vi "子VI-信息说明界面.vi"() -> ()   [LabVIEW 2018]
panel:
  in  "确认":bool
  out "使用说明":string
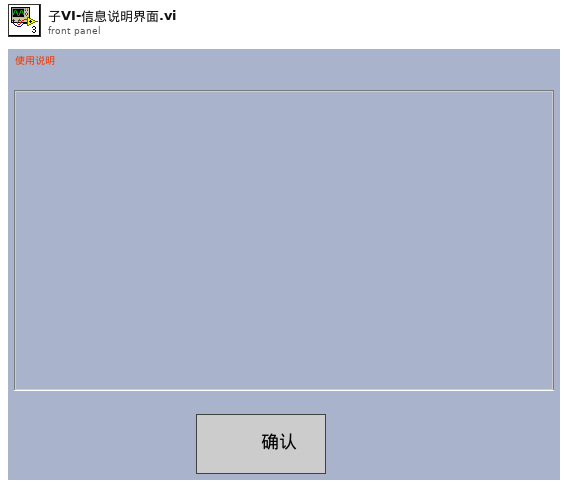
[diagram p1: front panel]
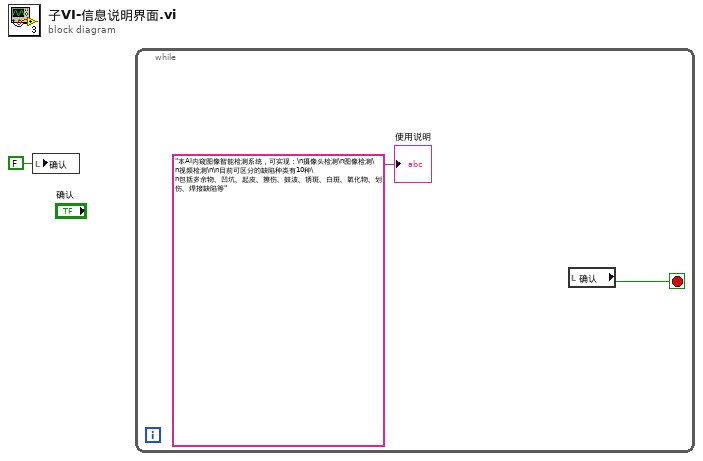
[diagram p0: block diagram]
diagram:
  n1 = local write "确认"(FALSE ("确定")) -> ()
  n2 = while {
    stop <- w2 stop-if-true
    n3 = local read "确认"() -> (w2:bool)
    "使用说明" <- "本AI内窥图像智能检测系统，可实现：\n摄像头检测\n图像检测\n视频检测\n\n目前可区分的缺陷种类有10种\n包括多余物、凹坑、起皮、擦伤、鼓波、锈斑、白斑、氧化物、划伤、焊接缺陷等" ("使用说明")
  }
